vi "highlightPlot.vi"(8 "error in (no error)":errorcluster, 10 "PlotNum":u32, 11 "QControl_Graph in":refnum<class "QControl_Graph.lvclass">) -> (0 "error out":errorcluster, 3 "QControl_Graph out":refnum<class "QControl_Graph.lvclass">)   [LabVIEW 2017, in "QControl_Graph.lvclass"]
uses:
  QControl_Graph.lvclass
  C:/Program Files (x86)/National Instruments/LabVIEW 2017/vi.lib/QSI/QControls/QControl Classes/WaveformGraph/WaveformGraph.lvclass
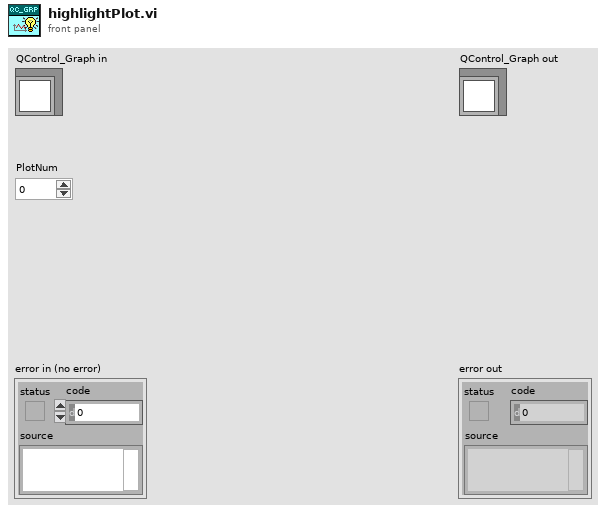
[diagram p1: front panel]
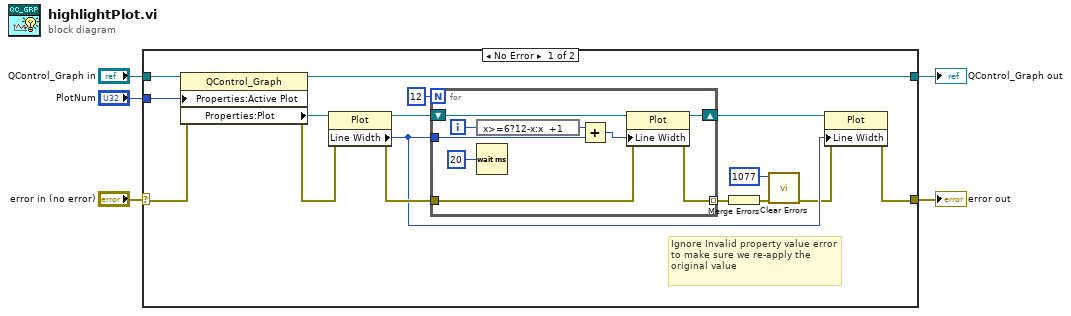
[diagram p0: block diagram]
diagram:
  n1 = case shown="No Error" "error in (no error)" {
    selector: "error in (no error)" -> [w11 w31]
    tunnel: [w20 w32] -> w3
    tunnel: "QControl_Graph in" -> [w21 w32]
    tunnel: "PlotNum" -> [w19 _]
    tunnel: [w9 w31] -> w1
    frame No Error {
      # "Ignore Invalid property value error to make sure we re-apply the original value"
      n2 = property class="QControl_Graph"(reference=w21, error in=w11, "Properties:Active Plot"=w19) -> (reference out=w20:refnum<class "QControl_Graph.lvclass">, error out=w12:errorcluster, "Properties:Plot"=w18:refnum<vi>)
      n3 = property class="Plot"(reference=w18, error in=w12) -> (reference out=w16:refnum<vi>, error out=w14:errorcluster, "Line Width"=w8:u8)
      n4 = for {
        N: 12 -> [_]
        tunnel: w8 -> [w27]
        shift-right: [w29] -> w15
        shift-left: w16 -> [w30]
        tunnel: w14 -> [w23]
        tunnel: [w22] -> w13 mode=indexing
        i -> [w28]
        n5 = expression code="x>=6?12-x:x  +1"(w28) -> (w25:i32)
        n6 = Wait (ms)(milliseconds to wait=u32 20) -> ()  [unwired: 1 out]
        n7 = Add(x=w25, y=w27) -> (x+y=w26:i32)
        n8 = property class="Plot"(reference=w30, error in=w23, "Line Width"=w26) -> (reference out=w29:refnum<vi>, error out=w22:errorcluster)
      }
      n9 = Merge Errors(w13) -> (w10:errorcluster)
      n10 = call <vilib>:"Clear Errors.vi"("error in (no error)"=w10, "specific error code to clear (0: all)"=1077) -> ("error out"=w7:errorcluster)  [unwired: 4 in, 1 out]
      n11 = property class="Plot"(reference=w15, error in=w7, "Line Width"=w8) -> (error out=w9:errorcluster)  [unwired: 1 out]
    }
    frame Error {
    }
  }
  "error out" <- w1
  "QControl_Graph out" <- w3
